vi "cont_array.vi"(11 "u8_ar_phase map":u8[](array[numeric])) -> (3 "Array":i16[](array[numeric]))   [LabVIEW 2011]
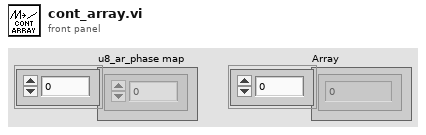
[diagram p1: front panel]
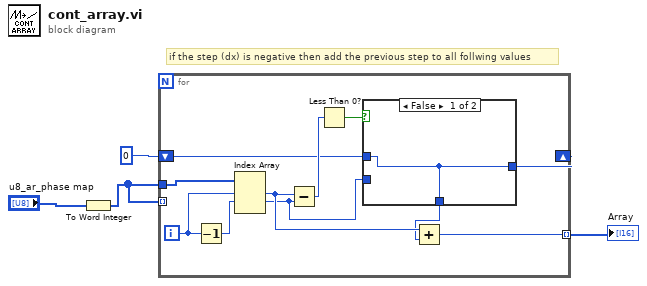
[diagram p0: block diagram]
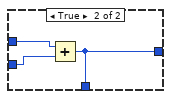
[diagram p2: hidden frame]
diagram:
  # "if the step (dx) is negative then add the previous step to all follwing values"
  n1 = To Word Integer(number="u8_ar_phase map") -> (16bit integer=w1:i16[])
  n2 = for {
    tunnel: w1 -> [w15]
    tunnel: w1 -> [_] mode=indexing
    shift-right: [w8] -> _
    shift-left: i16 0 -> [w7]
    tunnel: [w5] -> w3 mode=indexing
    i -> [w11]
    n3 = Decrement(x=w11) -> (x-1=w12:i32)
    n4 = Index Array(array=w15, index #1=w11, index #2=w12) -> (element #1=w10:i16, element #2=w9:i16)  [unwired: 1 in, 1 out]
    n5 = Subtract(x=w10, y=w9) -> (x-y=w14:i16)
    n6 = Less Than 0?(x=w14) -> (x < 0?=w13:bool)
    n7 = case shown="False" w13 {
      tunnel: w9 -> [_ w19]
      tunnel: [w16 w17] -> w8
      tunnel: w7 -> [w16 w18]
      tunnel: [w16 w17] -> w6
      frame False {
      }
      frame True {
        n8 = Add(x=w18, y=w19) -> (x+y=w17:i16)
      }
    }
    n9 = Add(x=w10, y=w6) -> (x+y=w5:i16)
  }
  "Array" <- w3
